vi "Run I2C Test.vi"(8 "error in (no error)":errorcluster, 10 "Position":u32, 11 "MTS I2C Test in":refnum<class "MTS I2C Test.lvclass">) -> (0 "error out":errorcluster, 3 "Passed":bool)   [LabVIEW 2015, in "MTS I2C Test.lvclass"]
uses:
  MTS I2C Test.lvclass
  <vilib>/Cree, Inc/Cree Test Framework/Core Launcher/Core Manager Methods -- Enum.ctl
  Classes/Instruments/I2C Device/NI-8452/Public API/Slave Wait on Event.vi
  Common RF Tests/RF Common Tests.lvclass
  Classes/Manufacturing Test/Class/SC Manufacturing Test.lvclass
  Classes/Instruments/I2C Device/NI-8452/NI-8452.lvclass
  <vilib>/Cree, Inc/Cree Test Framework/Classes/Base Objects/Base Class/Base Class/Base Class.lvclass
  <vilib>/Cree, Inc/Cree Test Framework/Classes/Data/Data Repo/Class/Data Repo.lvclass
  <vilib>/Cree, Inc/Cree Test Framework/Core Launcher/Core Launcher.lvlib
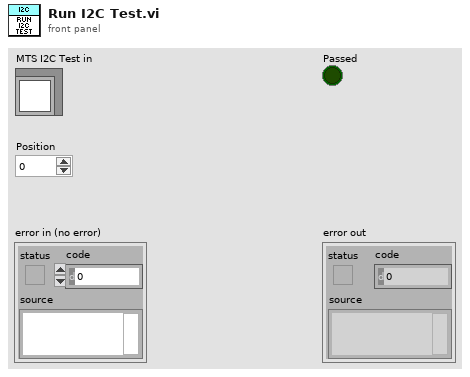
[diagram p1: front panel]
types:
  T1 = typedef "Core Launcher.lvlib/Core Manager Methods -- Enum.ctl" = enum16{"Spawn Objects", "Get Objects", "Destroy Objects"}
  T2 = typedef "ni845xI2cSlaveEventType.ctl" = enum8{"NoEvent", "CmdEvent", "DataAvailEvent", "DataReqEvent", "WriteCompleteEvent"}
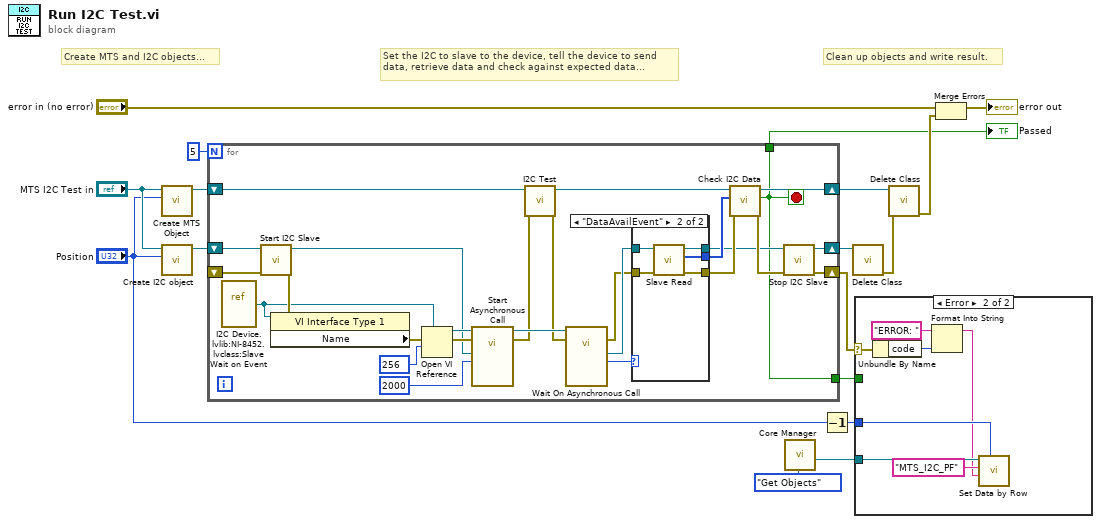
[diagram p0: block diagram]
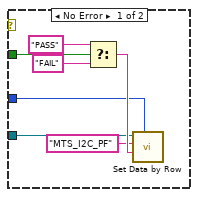
[diagram p2: hidden frame]
diagram:
  # "Clean up objects and write result."
  # "Set the I2C to slave to the device, tell the device to send data, retrieve data and check against expected data..."
  # "Create MTS and I2C objects..."
  n1 = call "Create MTS Object.vi"("Position"="Position", "RF Common Tests in"="MTS I2C Test in") -> ("SC Manufacturing Test out"=w14:refnum<class "SC Manufacturing Test.lvclass">)  [unwired: 8 in, 1 out]
  n2 = call "Create I2C object.vi"("Position"="Position", "MTS I2C Test in"="MTS I2C Test in") -> ("NI-8452 out"=w13:refnum<class "NI-8452.lvclass">)  [unwired: 8 in, 1 out]
  n3 = for {
    N: 5 -> [_]
    shift-right: [w24] -> w11
    shift-left: w14 -> [w39]
    shift-right: [w19] -> w12
    shift-left: w13 -> [w41]
    shift-right: [w21] -> w5
    shift-left: _ -> [w40]
    tunnel: [w18] -> w8
    tunnel: [w18] -> w1
    stop <- w18 stop-if-true
    n4 = vi-ref "I2C Device.lvlib:NI-8452.lvclass:Slave Wait on Event.vi"() -> (w38:refnum<vi>)
    n5 = call "Start I2C Slave.vi"("error in (no error)"=w40, "NI-8452 in"=w41) -> ("error out"=w42:errorcluster, "NI-8452 out"=w35:refnum<class "NI-8452.lvclass">)  [unwired: 8 in]
    n6 = property class="VI Interface Type 1"(reference=w38) -> ("Name"=w37:string)  [unwired: 1 in, 2 out]
    n7 = Open VI Reference(type specifier VI Refnum (for type only)=w38, vi path=w37, options=256) -> (vi reference=w36:refnum<vi>)  [unwired: 3 in, 1 out]
    n8 = call-by-ref "Start Asynchronous Call"(reference=w36, error in=w42, "Timeout (500ms)"=u32 2000, "NI-8452 in"=w35) -> (reference out=w33:refnum<vi>, error out=w32:errorcluster)  [unwired: 6 in, 4 out]
    n9 = call "I2C Test.vi"("error in (no error)"=w32, "Acrobat Template in"=w39) -> ("error out"=w31:errorcluster, "Acrobat Template out"=w27:refnum<class "SC Manufacturing Test.lvclass">)  [unwired: 8 in]
    n10 = call-by-ref "Wait On Asynchronous Call"(reference=w33, error in=w31) -> (error out=w29:errorcluster, "Event Type"=w28:T2, "NI-8452 out"=w30:refnum<class "NI-8452.lvclass">)  [unwired: 8 in, 3 out]
    n11 = case shown="\"DataAvailEvent\"" w28 {
      tunnel: w30 -> [w44 w49]
      tunnel: w29 -> [w43 w48]
      tunnel: [w44 w47] -> w20
      tunnel: [w43 w46] -> w25
      tunnel: [_ w45] -> w26
      frame Default {
      }
      frame "DataAvailEvent" {
        n12 = call "Slave Read.vi"("error in (no error)"=w48, "NI-8452 in"=w49) -> ("error out"=w46:errorcluster, "Data"=w45:u8[], "NI-8452 out"=w47:refnum<class "NI-8452.lvclass">)  [unwired: 7 in]
      }
    }
    n13 = call "Check I2C Data.vi"("error in (no error)"=w25, "Data"=w26, "Acrobat Template in"=w27) -> ("error out"=w22:errorcluster, "I2C Data Match"=w18:bool, "Acrobat Template out"=w24:refnum<class "SC Manufacturing Test.lvclass">)  [unwired: 6 in]
    n14 = call "Stop I2C Slave.vi"("error in (no error)"=w22, "NI-8452 in"=w20) -> ("error out"=w21:errorcluster, "NI-8452 out"=w19:refnum<class "NI-8452.lvclass">)  [unwired: 8 in]
  }
  "Passed" <- w1
  n15 = call <vilib>:"Core Manager.vi"("Method"=Core_Manager_Methods_--_Enum."Get Objects") -> ("Data Repo"=w9:refnum<class "Data Repo.lvclass">)  [unwired: 6 in, 4 out]
  n16 = Decrement(x="Position") -> (x-1=w6:u32)
  n17 = call <vilib>:"Delete Class.vi"("Base Class in"=w12) -> ("error out"=w10:errorcluster)  [unwired: 9 in, 1 out]
  n18 = case shown="Error" w5 {
    selector: w5 -> [_ w58]
    tunnel: w9 -> [w52 w62]
    tunnel: w8 -> [w51 _]
    tunnel: w6 -> [w50 w61]
    frame No Error {
      n19 = Select(t="PASS" ("Header"), s=w51, f="FAIL" ("Header")) -> (s? t:f=w55:string)
      n20 = call <vilib>:"Set Data by Row.vi"("Row"=w50, "Value"=w55, "Header"="MTS_I2C_PF", "Acrobat Template in"=w52) -> ()  [unwired: 6 in, 2 out]
    }
    frame Error {
      n21 = Unbundle By Name(w58) -> ("code"=w59:i32)
      n22 = Format Into String(initial string="ERROR: " ("Header"), w59) -> (resulting string=w57:string)  [unwired: 2 in, 1 out]
      n23 = call <vilib>:"Set Data by Row.vi"("Row"=w61, "Value"=w57, "Header"="MTS_I2C_PF", "Acrobat Template in"=w62) -> ()  [unwired: 6 in, 2 out]
    }
  }
  n24 = call <vilib>:"Delete Class.vi"("error in (no error)"=w10, "Base Class in"=w11) -> ("error out"=w3:errorcluster)  [unwired: 8 in, 1 out]
  n25 = Merge Errors("error in (no error)", w3) -> (→"error out":errorcluster)
